vi "PV ActiveLine - EndValue.vi"(7 "W/R":bool, 8 "Fehler (Eingang)":errorcluster, 9 "End Value":i8(ring) items=["UR/OR", "value"], 11 "Referenz in":refnum<visa-resource-name>) -> (0 "Cluster (Ausgang)":errorcluster, 1 "Read Status":u16(ring) items=["Read Failed", "Read Ok"], 2 "End Value Out":i8(ring) items=["UR/OR", "value"], 3 "Referenz out":refnum<visa-resource-name>)   [LabVIEW 2013, in "PV ActiveLine.lvlib"]
doc: "EVA - Measurement Range End Value\n\nTransmit: EVA [,a]\nReceive: a\n\nMeasurement range end value,\na =\n0 –> UR or OR is displayed (default) when an underrange or overrange occurs\n1 –> The measurement range end value is displayed when an underrange or overrange occurs"
uses:
  <instrlib>/PV ActiveLine/PV ActiveLine.lvlib
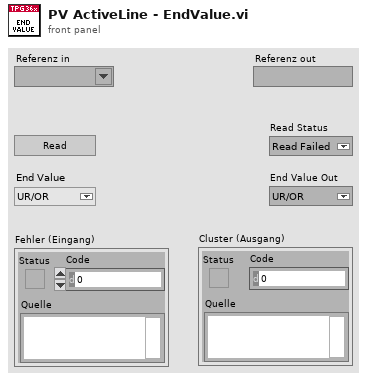
[diagram p1: front panel]
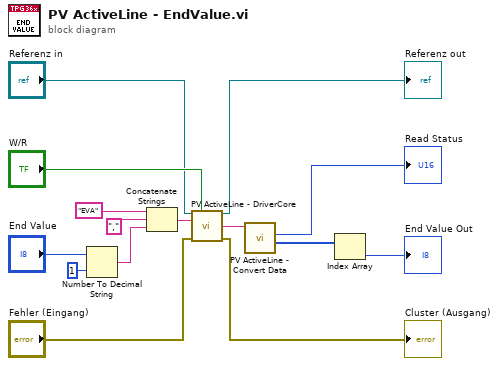
[diagram p0: block diagram]
diagram:
  n1 = Number To Decimal String(number="End Value", width (-)=i16 1) -> (decimal integer string=w12:string)
  n2 = Concatenate Strings("EVA" ("Command"), "," ("Command"), w12) -> (w9:string)
  n3 = call <instrlib>:"PV ActiveLine - DriverCore.vi"("Referenz in"="Referenz in", "Write/Read"="W/R", "Command"=w9, "Fehler (Eingang)"="Fehler (Eingang)") -> ("Referenz out"=→"Referenz out":refnum<visa-resource-name>, "String Out"=w4:string, "Cluster (Ausgang)"=→"Cluster (Ausgang)":errorcluster)  [unwired: 9 in]
  n4 = call <instrlib>:"PV ActiveLine - Convert Data.vi"("String in"=w4) -> ("Integer Out"=w3:i32[], "Read Status"=→"Read Status":u16)  [unwired: 7 in, 2 out]
  n5 = Index Array(array=w3) -> (element=→"End Value Out":i32)  [unwired: 1 in]
